vi "After Launch Init Core.vi"(8 "error in (no error)":errorcluster, 11 "CS++DCPwr in":refnum<class "CS++DCPwr.lvclass">) -> (0 "error out":errorcluster, 3 "CS++DCPwr out":refnum<class "CS++DCPwr.lvclass">)   [LabVIEW 2015, in "CS++DCPwr.lvlib" / "CS++DCPwr.lvclass"]
doc: "Use <b>Pre Launch init.vi</b> method for sanity checks that are supposed to prevent the actor from launching if they fail. Use <B>this</B> method instead to initialize this actor when it has been activated. A corresponding high priority message will become dispatched before the <B>Actor Core.vi</b> is called.\n\nRefer also to the ongoing discussion at https://decibel.ni.com/content/message/57394#57394."
uses:
  CS++DCPwr.lvclass
  CSPP_Core/Classes/CS++ProcessVariables/ProcessVariable/PV.lvclass
  CS++DCPwr.lvclass/CS++DCPwr.ctl
  CSPP_Core/Classes/CS++ProcessVariables/ProcessVariable/PV.lvclass/PV.ctl
  CSPP_Core/Actors/CS++BaseActor/CS++BaseActor.lvclass/CS++BaseActor.ctl
  CS++DCPwr Messages/Measure [MSR] Msg/Measure [MSR] Msg.lvclass
  <vilib>/ActorFramework/Actor/Actor.lvclass/Actor.ctl
  <vilib>/ActorFramework/Message Enqueuer/Message Enqueuer.lvclass/Message Enqueuer.ctl
  CS++DCPwr Messages/Measure [MSR] Msg/Measure [MSR] Msg.lvclass/Measure [MSR] Msg.ctl
  CS++DCPwr Messages/Measure [MSR] Msg/Write channel name.vi
  CS++DCPwr Messages/Measure [MSR] Msg/Write measurement type.vi
  CSPP_Core/Classes/CS++ProcessVariables/ProcessVariable/Write Data.vi
  CSPP_Core/Classes/CS++ProcessVariables/ProcessVariable/Write Error.vi
  CSPP_Core/Classes/CS++ProcessVariables/ProcessVariable/Write Quality.vi
  CSPP_Core/Classes/CS++ProcessVariables/ProcessVariable/Write status.vi
  CSPP_Core/Classes/CS++ProcessVariables/ProcessVariable/Write Timestamp.vi
  <vilib>/ActorFramework/Message Enqueuer/Init from Existing Queue.vi
  <vilib>/ActorFramework/Message Enqueuer/Message Enqueuer.lvclass
  CSPP_Core/Actors/CS++DeviceActor/CS++DeviceActor.lvclass
  <vilib>/ActorFramework/Actor/Actor.lvclass
  CSPP_Core/Actors/CS++BaseActor/CS++BaseActor.lvclass
  CSPP_Core/Classes/CS++ProcessVariables/PVConnection/PVConnection.lvclass
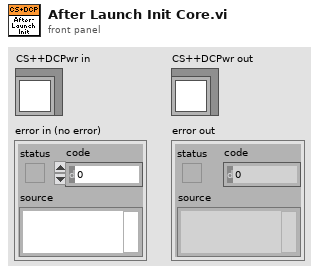
[diagram p1: front panel]
types:
  T1 = cluster{"Read Access":enum8{"Allowed", "Required", "None"}, "Write Access":enum8{"Allowed", "Required", "None"}}
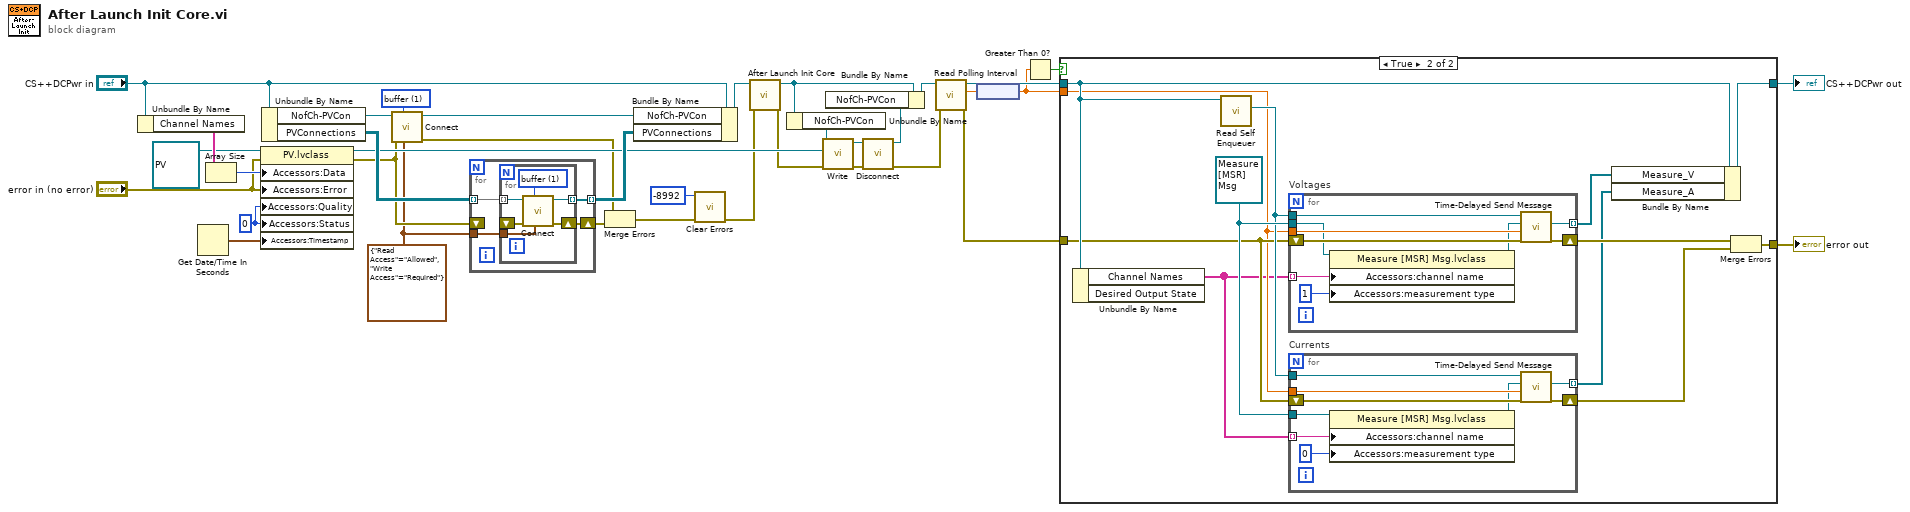
[diagram p0: block diagram]
diagram:
  w12 = u16 1 items=["commit", "buffer"] ("Mode (commit)")
  w14 = T1 {"Read Access"=enum."Allowed", "Write Access"=enum."Required"} ("Access (R/W allowed)")
  w24 = 0 ("Quality")
  n1 = Unbundle By Name("CS++DCPwr in") -> ("Channel Names"=w28:string[])
  n2 = Get Date/Time In Seconds() -> (seconds since 1Jan1904=w23:timestamp)
  n3 = Array Size(array=w28) -> (size(s)=w26:i32)
  n4 = property class="PV.lvclass"(reference=refnum<class "PV.lvclass"> refnum ("CS++ProcessVariables.lvlib:PV.lvclass"), error in="error in (no error)", "Accessors:Data"=w26, "Accessors:Error"="error in (no error)", "Accessors:Quality"=w24, "Accessors:Status"=w24, "Accessors:Timestamp"=w23) -> (reference out=w16:refnum<class "PV.lvclass">, error out=w15:errorcluster)
  n5 = Unbundle By Name("CS++DCPwr in") -> ("NofCh-PVCon"=w19:refnum<class "PVConnection.lvclass">, "PVConnections"=w21:refnum<class "PVConnection.lvclass">[][])
  n6 = call "Connect.vi"("Access (R/W allowed)"=w14, "Mode (buffer)"=w12, "Error In"=w15, "PVConnection in"=w19) -> ("Error Out"=w9:errorcluster, "PVConnection out"=w5:refnum<class "PVConnection.lvclass">)  [unwired: 6 in]
  n7 = for {
    tunnel: w14 -> [w40]
    tunnel: w21 -> [w39] mode=indexing
    tunnel: [w38] -> w20 mode=indexing
    shift-right: [w37] -> w8
    shift-left: w15 -> [_]
    n8 = for {
      tunnel: w39 -> [w46] mode=indexing
      tunnel: [w45] -> w38 mode=indexing
      tunnel: w40 -> [w44]
      shift-right: [w43] -> w37
      shift-left: _ -> [w42]
      w41 = u16 1 items=["commit", "buffer"] ("Mode (commit)")
      n9 = call "Connect.vi"("Access (R/W allowed)"=w44, "Mode (buffer)"=w41, "Error In"=w42, "PVConnection in"=w46) -> ("Error Out"=w43:errorcluster, "PVConnection out"=w45:refnum<class "PVConnection.lvclass">)  [unwired: 6 in]
    }
  }
  n10 = Merge Errors(w9, w8) -> (w7:errorcluster)
  n11 = Bundle By Name(cluster="CS++DCPwr in", "NofCh-PVCon"=w5, "PVConnections"=w20) -> (w36:refnum<class "CS++DCPwr.lvclass">)
  n12 = call <vilib>:"Clear Errors.vi"("error in (no error)"=w7, "specific error code to clear (0: all)"=-8992) -> ("error out"=w6:errorcluster)  [unwired: 4 in, 1 out]
  n13 = call-parent "After Launch Init Core.vi"("error in (no error)"=w6, "CS++DeviceActor in"=w36) -> ("error out"=w2:errorcluster, "CS++DeviceActor out"=w11:refnum<class "CS++DCPwr.lvclass">)  [unwired: 8 in]
  n14 = Unbundle By Name(w11) -> ("NofCh-PVCon"=w4:refnum<class "PVConnection.lvclass">)
  n15 = call "Write.vi"("error in (no error)"=w2, "PV"=w16, "PVConnection in"=w4) -> ("error out"=w17:errorcluster, "PVConnection out"=w18:refnum<class "PVConnection.lvclass">)  [unwired: 7 in]
  n16 = call "Disconnect.vi"("error in (no error)"=w17, "PVConnection in"=w18) -> ("error out"=w1:errorcluster, "PVConnection out"=w3:refnum<class "PVConnection.lvclass">)  [unwired: 8 in]
  n17 = Bundle By Name(cluster=w11, "NofCh-PVCon"=w3) -> (w10:refnum<class "CS++DCPwr.lvclass">)
  n18 = call "Read Polling Interval.vi"("error in (no error)"=w1, "CS++BaseActor in"=w10) -> ("error out"=w34:errorcluster, "Polling Interval"=w33:dbl[unit], "CS++BaseActor out"=w35:refnum<class "CS++DCPwr.lvclass">)  [unwired: 7 in]
  n19 = node(w33) -> (w32:dbl)
  n20 = Greater Than 0?(x=w32) -> (x > 0?=w31:bool)
  n21 = case shown="True" w31 {
    tunnel: [w48 w60] -> w30
    tunnel: [w47 w58] -> w29
    tunnel: w35 -> [w48 w59]
    tunnel: w34 -> [w47 w51]
    tunnel: w32 -> [_ w50]
    frame False {
    }
    frame True {
      w53 = refnum<class "Measure [MSR] Msg.lvclass"> refnum ("CS++DCPwr.lvlib:Measure [MSR] Msg.lvclass")
      n22 = Unbundle By Name(w59) -> ("Channel Names"=w49:string[])  [unwired: 1 out]
      n23 = call <vilib>:"Read Self Enqueuer.vi"("Actor"=w59) -> ("Self Enqueuer"=w52:refnum<class "Message Enqueuer.lvclass">)  [unwired: 10 in]
      n24 = for "Voltages" {
        tunnel: w52 -> [w77]
        tunnel: w50 -> [w75]
        tunnel: [w74] -> w56 mode=indexing
        tunnel: w53 -> [w70]
        shift-right: [w78] -> w57
        shift-left: w51 -> [w76]
        tunnel: w49 -> [w73] mode=indexing
        n25 = property class="Measure [MSR] Msg.lvclass"(reference=w70, "Accessors:channel name"=w73, "Accessors:measurement type"=1 ("measurement type (voltage)")) -> (reference out=w71:refnum<class "Measure [MSR] Msg.lvclass">)  [unwired: 1 in, 1 out]
        n26 = call <vilib>:"Time-Delayed Send Message.vi"("error in (no error)"=w76, "Milliseconds To Wait"=w75, "Message"=w71, "Message Enqueuer"=w77) -> ("error out"=w78:errorcluster, "Delivery Notifier"=w74:refnum<notifier>)  [unwired: 6 in]
      }
      n27 = for "Currents" {
        tunnel: w52 -> [w68]
        tunnel: w50 -> [w66]
        tunnel: [w65] -> w55 mode=indexing
        shift-right: [w69] -> w54
        shift-left: w51 -> [w67]
        tunnel: w49 -> [w64] mode=indexing
        tunnel: w53 -> [w61]
        n28 = property class="Measure [MSR] Msg.lvclass"(reference=w61, "Accessors:channel name"=w64, "Accessors:measurement type"=0 ("measurement type (voltage)")) -> (reference out=w62:refnum<class "Measure [MSR] Msg.lvclass">)  [unwired: 1 in, 1 out]
        n29 = call <vilib>:"Time-Delayed Send Message.vi"("error in (no error)"=w67, "Milliseconds To Wait"=w66, "Message"=w62, "Message Enqueuer"=w68) -> ("error out"=w69:errorcluster, "Delivery Notifier"=w65:refnum<notifier>)  [unwired: 6 in]
      }
      n30 = Bundle By Name(cluster=w59, "Measure_V"=w56, "Measure_A"=w55) -> (w60:refnum<class "CS++DCPwr.lvclass">)
      n31 = Merge Errors(w57, w54) -> (w58:errorcluster)
    }
  }
  "error out" <- w29
  "CS++DCPwr out" <- w30
